vi "ex2.vi"() -> ()   [LabVIEW 2022 SP3]
panel:
  in  "Font Size":i32
  in  "Color Box":u32(colorbox)
  in  "Text":string
  in  "Underline":bool
  in  "Cursive":bool
  in  "Bold":bool
  in  "stop":bool
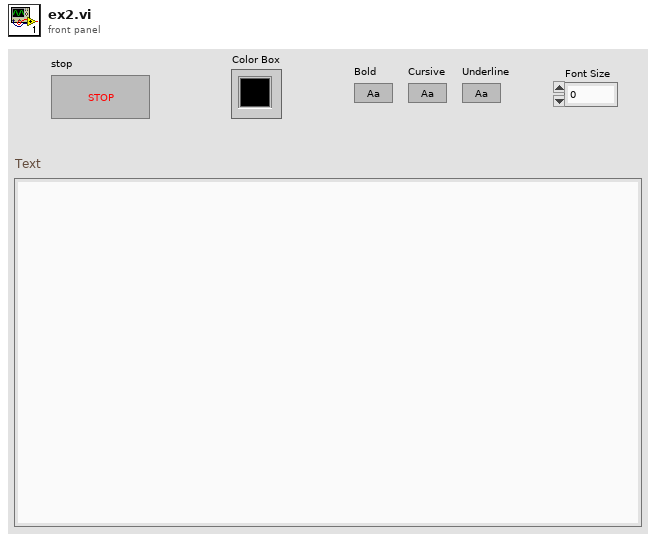
[diagram p1: front panel]
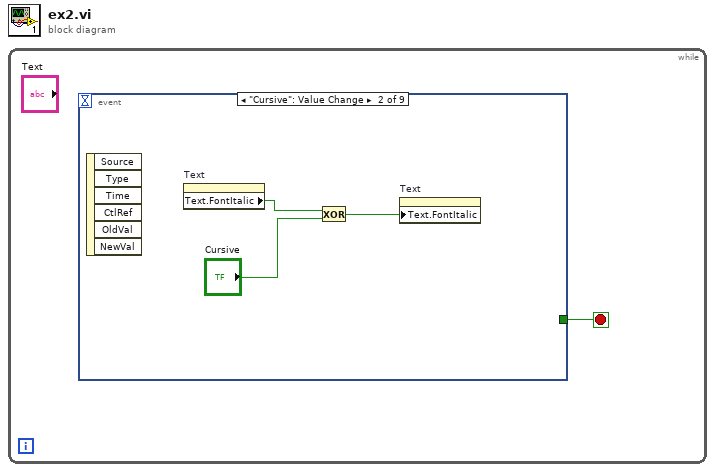
[diagram p0: block diagram]
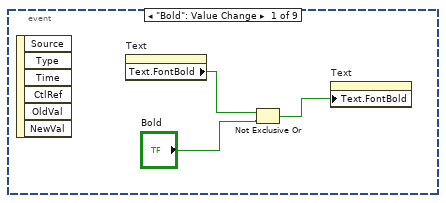
[diagram p2: hidden frame]
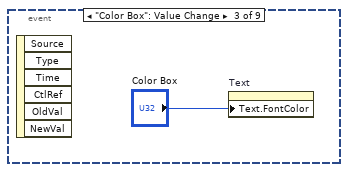
[diagram p3: hidden frame]
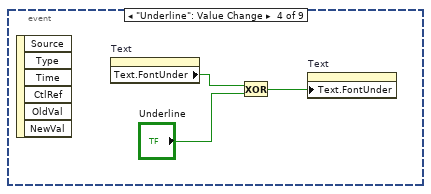
[diagram p4: hidden frame]
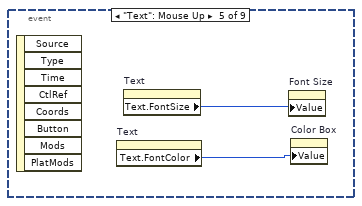
[diagram p5: hidden frame]
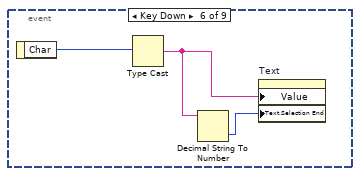
[diagram p6: hidden frame]
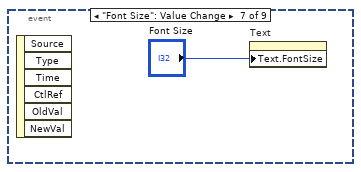
[diagram p7: hidden frame]
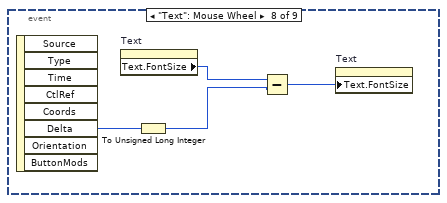
[diagram p8: hidden frame]
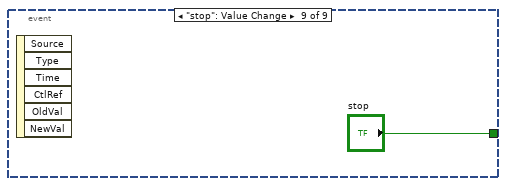
[diagram p9: hidden frame]
diagram:
  n1 = while {
    stop <- w1 stop-if-true
    n2 = event shown="[1] \"Cursive\": Value Change" {
      selector: _ -> [_ _ _ _ _ _ _ _ _]
      dyn-events: _ -> [_ _ _ _ _ _ _ _ _]
      timeout: _ -> [_ _ _ _ _ _ _ _ _]
      tunnel: [_ _ _ _ _ _ _ _ "stop"] -> w1
      event "Bold": Value Change {
        n3 = event-data() -> ()  [unwired: 1 in, 6 out]
        n4 = property on="Text" class="Str"() -> ("Text.FontBold"=w4:bool)  [unwired: 2 in, 2 out]
        n5 = Not Exclusive Or(1:"Bold", 2:w4) -> (0:w2:bool)
        n6 = property on="Text" class="Str"("Text.FontBold"=w2) -> ()  [unwired: 2 in, 2 out]
      }
      event "Cursive": Value Change {
        n7 = event-data() -> ()  [unwired: 1 in, 6 out]
        n8 = property on="Text" class="Str"() -> ("Text.FontItalic"=w7:bool)  [unwired: 2 in, 2 out]
        n9 = Exclusive Or(1:"Cursive", 2:w7) -> (0:w5:bool)
        n10 = property on="Text" class="Str"("Text.FontItalic"=w5) -> ()  [unwired: 2 in, 2 out]
      }
      event "Color Box": Value Change {
        n11 = event-data() -> ()  [unwired: 1 in, 6 out]
        n12 = property on="Text" class="Str"("Text.FontColor"="Color Box") -> ()  [unwired: 2 in, 2 out]
      }
      event "Underline": Value Change {
        n13 = event-data() -> ()  [unwired: 1 in, 6 out]
        n14 = property on="Text" class="Str"() -> ("Text.FontUnder"=w11:bool)  [unwired: 2 in, 2 out]
        n15 = Exclusive Or(1:"Underline", 2:w11) -> (0:w9:bool)
        n16 = property on="Text" class="Str"("Text.FontUnder"=w9) -> ()  [unwired: 2 in, 2 out]
      }
      event "Text": Mouse Up {
        n17 = event-data() -> ()  [unwired: 1 in, 8 out]
        n18 = property on="Text" class="Str"() -> ("Text.FontColor"=w12:u32)  [unwired: 2 in, 2 out]
        n19 = property on="Text" class="Str"() -> ("Text.FontSize"=w13:u32)  [unwired: 2 in, 2 out]
        n20 = property on="Font Size" class="DigNum (strict)"("Value"=w13) -> ()  [unwired: 2 in, 2 out]
        n21 = property on="Color Box" class="ColBox"("Value"=w12) -> ()  [unwired: 2 in, 2 out]
      }
      event Key Down {
        n22 = event-data() -> ("Char"=w16:i16)  [unwired: 1 in]
        n23 = Type Cast(x=w16) -> (*(type *) &x=w15:string)  [unwired: 1 in]
        n24 = Decimal String To Number(string=w15) -> (number=w14:i32)  [unwired: 2 in, 1 out]
        n25 = property on="Text" class="Str"("Value"=w15, "Text.Selection End"=w14) -> ()  [unwired: 2 in, 2 out]
      }
      event "Font Size": Value Change {
        n26 = event-data() -> ()  [unwired: 1 in, 6 out]
        n27 = property on="Text" class="Str"("Text.FontSize"="Font Size") -> ()  [unwired: 2 in, 2 out]
      }
      event "Text": Mouse Wheel {
        n28 = event-data() -> ("Delta"=w21:i32)  [unwired: 1 in, 7 out]
        n29 = property on="Text" class="Str"() -> ("Text.FontSize"=w20:u32)  [unwired: 2 in, 2 out]
        n30 = To Unsigned Long Integer(number=w21) -> (unsigned 32bit integer=w19:u32)
        n31 = Subtract(x=w20, y=w19) -> (x-y=w18:u32)
        n32 = property on="Text" class="Str"("Text.FontSize"=w18) -> ()  [unwired: 2 in, 2 out]
      }
      event "stop": Value Change {
        n33 = event-data() -> ()  [unwired: 1 in, 6 out]
      }
    }
  }
